vi "Pass If Matches Regular Expression.vi"(7 "Show \\ codes (F)":bool, 8 "error in (no error)":errorcluster, 9 "actual":string, 10 "regular expression":string, 11 "TestCase in":refnum<class "TestCase.lvclass">) -> (0 "error out":errorcluster, 3 "TestCase out":refnum<class "TestCase.lvclass">)   [LabVIEW 2015, in "VITAC.lvlib"]
doc: "Compares a string to a regular expression and passes if it matches. This VI uses the same PCRL regular expressions as the matches pattern VI.\n\nThe results string will include the full string and regex if it fails. You can use the <b>Show \\ codes</b> input to use the backslash codes in the string output."
uses:
  VITAC.lvlib
  <vilib>/addons/_JKI Toolkits/VI Tester/TestCase.llb/TestCase.lvclass
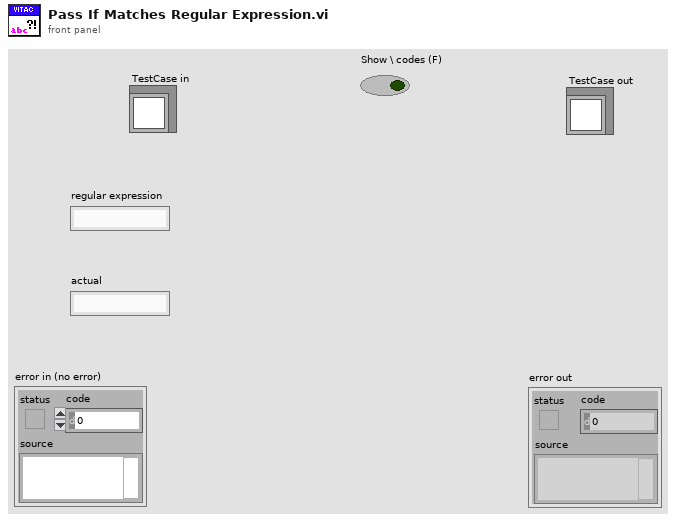
[diagram p1: front panel]
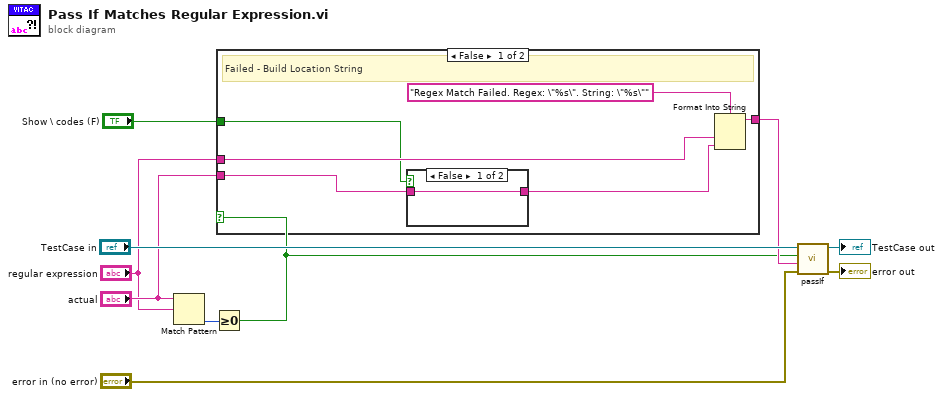
[diagram p0: block diagram]
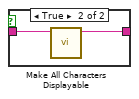
[diagram p2: hidden frame]
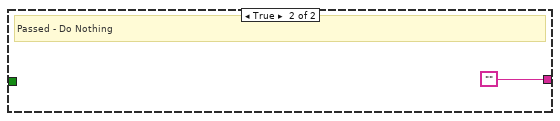
[diagram p3: hidden frame]
diagram:
  n1 = Match Pattern(string="actual", regular expression="regular expression") -> (offset past match=w3:i32)  [unwired: 1 in, 3 out]
  n2 = Greater Or Equal To 0?(x=w3) -> (x >= 0?=w2:bool)
  n3 = case shown="False" w2 {
    tunnel: "regular expression" -> [w13 _]
    tunnel: "actual" -> [w14 _]
    tunnel: [w15 ""] -> w6
    tunnel: "Show \\ codes (F)" -> [w11 _]
    frame False {
      # "Failed - Build Location String"
      n4 = case shown="False" w11 {
        tunnel: w14 -> [w17 w19]
        tunnel: [w17 w18] -> w12
        frame False {
        }
        frame True {
          n5 = call "Make All Characters Displayable.vi"("String In"=w19) -> ("Escaped String"=w18:string)  [unwired: 10 in]
        }
      }
      n6 = Format Into String(format string="Regex Match Failed. Regex: \"%s\". String: \"%s\"", w13, w12) -> (resulting string=w15:string)  [unwired: 2 in, 1 out]
    }
    frame True {
      # "Passed - Do Nothing"
    }
  }
  n7 = call-dynamic "passIf.vi"("error in (no error)"="error in (no error)", "message (\"\")"=w6, "pass"=w2, "TestCase in"="TestCase in") -> ("error out"=→"error out":errorcluster, "TestCase out"=→"TestCase out":refnum<class "TestCase.lvclass">)  [unwired: 6 in]
